vi "Decrement Twitter Max ID.vi"(8 "error in (no error)":errorcluster, 11 "ID In":string) -> (0 "error out":errorcluster, 3 "ID Out":string)   [LabVIEW 2011, in "i3-twitter.lvlib"]
doc: "Decrease string ID by one"
uses:
  i3-twitter.lvlib
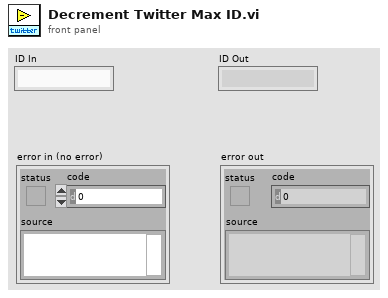
[diagram p1: front panel]
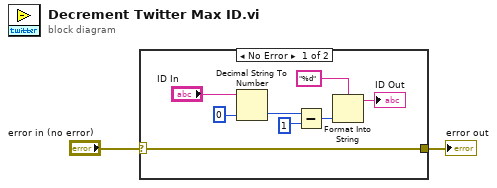
[diagram p0: block diagram]
diagram:
  n1 = case shown="No Error" "error in (no error)" {
    selector: "error in (no error)" -> [w3 w11]
    tunnel: [w3 w11] -> w1
    frame No Error {
      n2 = Decimal String To Number(string="ID In", default (0L)=i64 0 ("default (0 I32)")) -> (number=w6:i64)  [unwired: 1 in, 1 out]
      n3 = Subtract(x=w6, y=i64 1) -> (x-y=w8:i64)
      n4 = Format Into String(format string="%d", w8) -> (resulting string=→"ID Out":string)  [unwired: 2 in, 1 out]
    }
    frame Error {
    }
  }
  "error out" <- w1
